vi "VI Invoke Node-placeContent.vi"   [LabVIEW 2017]
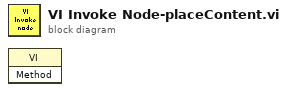
[diagram p0: block diagram]
diagram:
  n1 = invoke class="VI" method=#-1() -> ()  [unwired: 3 in, 3 out]
